vi "Distance to next node.vi"(10 "Nodes":cluster{i32, i32}[](array[cluster]), 11 "Grid":bool[][](array[boolean])) -> (3 "Next Node Map":T1(c390))   [LabVIEW 2021]
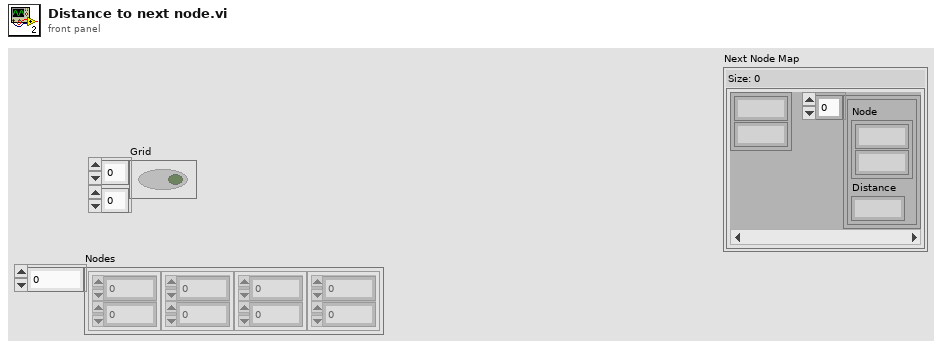
[diagram p1: front panel]
types:
  T1 = map{cluster{i32, i32}, cluster{"Node":cluster{i32, i32}, "Distance":i64}[]}
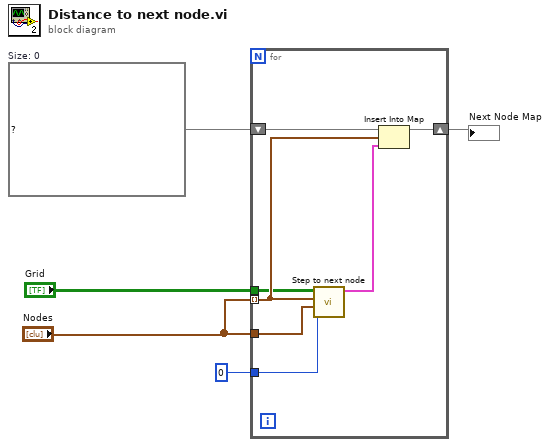
[diagram p0: block diagram]
diagram:
  w3 = T1 {}  # Size: 0
  n1 = for {
    tunnel: "Nodes" -> [w9] mode=indexing
    tunnel: "Grid" -> [w8]
    tunnel: "Nodes" -> [w10]
    shift-right: [w11] -> w2
    shift-left: w3 -> [w12]
    tunnel: 0 -> [w6]
    n2 = call "Step to next node.vi"("Numeric"=w6, "Nodes"=w10, "Cluster"=w9, "Grid"=w8) -> ("Distance to next node"=w7:cluster{cluster{i32, i32}, i32}[])  [unwired: 7 in]
    n3 = Insert Into Map(map in=w12, key=w9, value=w7) -> (map out=w11:T1)  [unwired: 2 out]
  }
  "Next Node Map" <- w2
